vi "Convert Tag List to CVT Tags.vi"(11 "CCC tag list":T3[](array[typedef])) -> (3 "CVT tag list":T1[](array[typedef]))   [LabVIEW 2010, in "NI_CCC.lvlib"]
uses:
  NI_CCC.lvlib
  Tag Configuration.ctl
  <vilib>/NI/Current Value Table/Type Defs/Data Types.ctl
  Tag Direction.ctl
  <vilib>/NI/Current Value Table/Type Defs/Single Tag.ctl
  <vilib>/NI/Current Value Table/Current Value Table.lvlib
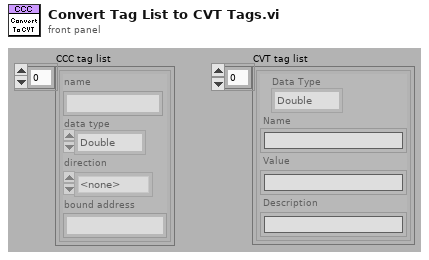
[diagram p1: front panel]
types:
  T1 = typedef "Current Value Table.lvlib/Single Tag.ctl" = cluster{"Data Type":T2, "Name":string, "Value":string, "Description":string}
  T2 = typedef "Current Value Table.lvlib/Data Types.ctl" = enum16{"Double", "Single", "I64", "I32", "I16", "I8", "U64", "U32", "U16", "U8", "String", "Boolean", "Array of U8", "Array of U16", "Array of U32", "Array of U64", "Array of I64", "Array of I32", "Array of I16", "Array of I8", "Array of Double", "Array of Single", "Array of Boolean", "Array of String"}
  T3 = typedef "NI_CCC.lvlib/Tag Configuration.ctl" = cluster{"name":string, "data type":T2, "direction":T4, "bound address":string}
  T4 = typedef "NI_CCC.lvlib/Tag Direction.ctl" = enum32{"<none>", "Read", "Write"}
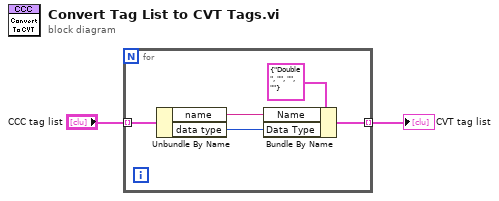
[diagram p0: block diagram]
diagram:
  n1 = for {
    tunnel: "CCC tag list" -> [w7] mode=indexing
    tunnel: [w3] -> w1 mode=indexing
    n2 = Unbundle By Name(w7) -> ("name"=w5:string, "data type"=w4:T2)
    n3 = Bundle By Name(cluster=T1 {"Data Type"=enum."Double", "Name"="", "Value"="", "Description"=""} ("Tag"), "Name"=w5, "Data Type"=w4) -> (w3:T1)
  }
  "CVT tag list" <- w1
